vi "Drive_AutoShift.vi"(5 "Max":dbl format="%#_13g", 6 "Force Low Gear":bool, 7 "ShifterRef":T2={"DevStatus"={"status"=FALSE, "code"=0, "source"=""}, "Pneumatics Control Module"=0, "Forward Solenoid Channel"=enum."Invalid", "Reverse Solenoid Channel"=enum."Invalid"}, 8 "Right  Input":dbl, 9 "Left Input":dbl, 10 "Right RPM":dbl, 11 "Left RPM":dbl) -> (1 "Shifting":bool, 2 "Right Output":dbl, 3 "Left Output":dbl, 4 "Gear":T1)   [LabVIEW 2016]
uses:
  <vilib>/Rock Robotics/WPI/Solenoid/WPI_SolenoidDevRef.ctl
  <vilib>/Rock Robotics/WPI/Solenoid/WPI_SolenoidChannel.ctl
  <vilib>/Rock Robotics/WPI/Solenoid/WPI_SolenoidValue.ctl
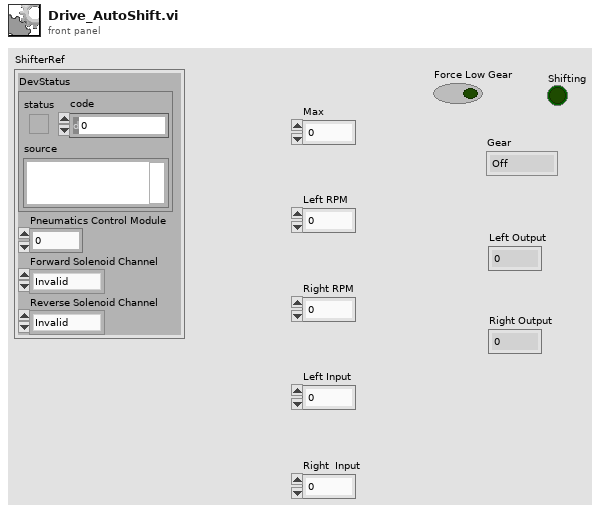
[diagram p1: front panel]
types:
  T1 = typedef "WPI_SolenoidValue.ctl" = enum16{"Off", "On", "Forward", "Reverse"}
  T2 = typedef "WPI_SolenoidDevRef.ctl" = cluster{"DevStatus":errorcluster, "Pneumatics Control Module":u8, "Forward Solenoid Channel":T3, "Reverse Solenoid Channel":T3}
  T3 = typedef "WPI_SolenoidChannel.ctl" = enum8{"Solenoid 0", "Solenoid 1", "Solenoid 2", "Solenoid 3", "Solenoid 4", "Solenoid 5", "Solenoid 6", "Solenoid 7", "Invalid"}
  T4 = cluster{"OutputMAX":dbl, "OutputMIN":dbl, "InputMAX":dbl, "InputMIN":dbl}
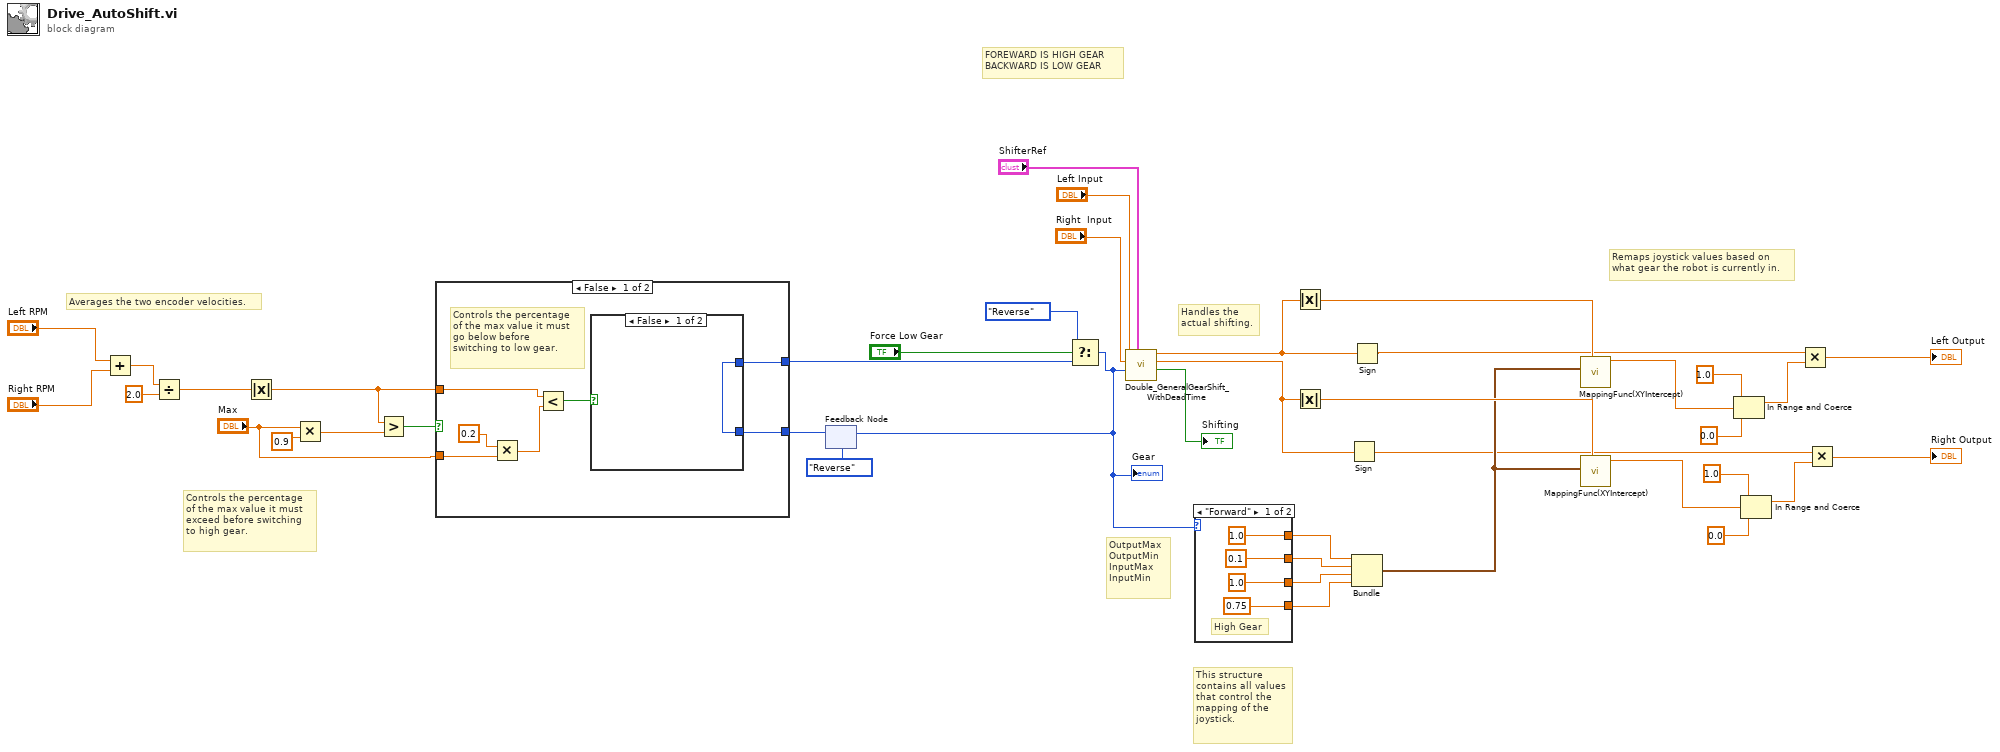
[diagram p0: block diagram]
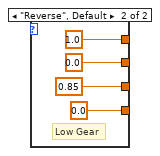
[diagram p2: hidden frame]
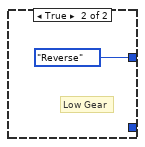
[diagram p3: hidden frame]
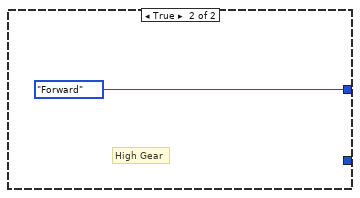
[diagram p4: hidden frame]
diagram:
  # "OutputMax\nOutputMin\nInputMax\nInputMin"
  # "This structure\ncontains all values\nthat control the\nmapping of the \njoystick."
  # "Remaps joystick values based on\nwhat gear the robot is currently in."
  # "Handles the\nactual shifting."
  # "FOREWARD IS HIGH GEAR\nBACKWARD IS LOW GEAR"
  # "Controls the percentage\nof the max value it must \nexceed before switching\nto high gear."
  # "Averages the two encoder velocities."
  n1 = Add(x="Left RPM", y="Right RPM") -> (x+y=w30:dbl)
  n2 = Divide(x=w30, y=2.0) -> (x/y=w7:dbl)
  n3 = Absolute Value(x=w7) -> (abs(x)=w6:dbl)
  n4 = Multiply(x="Max", y=0.9) -> (x*y=w40:dbl)
  n5 = Greater?(x=w6, y=w40) -> (0:w39:bool)
  n6 = feedback #1(WPI_SolenoidValue."Reverse" ("Shift Value")) -> (w3:T1)
  n7 = case shown="False" w39 {
    tunnel: [w44 WPI_SolenoidValue."Forward" ("Shift Value")] -> w21
    tunnel: "Max" -> [w47 _]
    tunnel: w3 -> [w43 _]
    tunnel: w6 -> [w42 _]
    frame False {
      # "Controls the percentage\nof the max value it must \ngo below before \nswitching to low gear."
      n8 = Multiply(x=0.2, y=w47) -> (x*y=w45:dbl)
      n9 = Less?(x=w42, y=w45) -> (x < y?=w48:bool)
      n10 = case shown="False" w48 {
        tunnel: [w49 WPI_SolenoidValue."Reverse" ("Shift Value")] -> w44
        tunnel: w43 -> [w49 _]
        frame False {
        }
        frame True {
          # "Low Gear"
        }
      }
    }
    frame True {
      # "High Gear"
    }
  }
  n11 = Select(t=WPI_SolenoidValue."Reverse", s="Force Low Gear", f=w21) -> (s? t:f=w2:T1)
  "Gear" <- w2
  n12 = feedback-in #1(w2) -> ()
  n13 = call "Double_GeneralGearShift_WithDeadTime.vi"("ShifterRef"="ShifterRef", "Shift Value"=w2, "Right"="Right  Input", "Left"="Left Input") -> ("Shifting"=→"Shifting":bool, "Right Output"=w15:dbl, "Left Output"=w13:dbl)  [unwired: 4 in, 1 out]
  n14 = case shown="\"Forward\"" w2 {
    tunnel: [1.0 ("OutputMAX") 1.0 ("OutputMAX")] -> w18
    tunnel: [0.1 ("OutputMIN") 0.0 ("OutputMIN")] -> w17
    tunnel: [1.0 ("InputMAX") 0.85 ("InputMAX")] -> w19
    tunnel: [0.75 ("InputMIN") 0.0 ("InputMIN")] -> w20
    frame "Forward" {
      # "High Gear"
    }
    frame "Reverse", Default {
      # "Low Gear"
    }
  }
  n15 = Absolute Value(x=w13) -> (abs(x)=w35:dbl)
  n16 = Absolute Value(x=w15) -> (abs(x)=w25:dbl)
  n17 = Sign(1:w15) -> (0:w14:dbl)
  n18 = Sign(1:w13) -> (0:w12:dbl)
  n19 = Bundle("OutputMAX"=w18, "OutputMIN"=w17, "InputMAX"=w19, "InputMIN"=w20) -> (w16:T4)  [unwired: 1 in]
  n20 = call "MappingFunc(XYIntercept).vi"("Input"=w35, "Cluster"=w16) -> ("Output"=w34:dbl)  [unwired: 9 in]
  n21 = call "MappingFunc(XYIntercept).vi"("Input"=w25, "Cluster"=w16) -> ("Output"=w26:dbl)  [unwired: 9 in]
  n22 = In Range and Coerce(upper limit=1.0, x=w34, lower limit=0.0) -> (coerced(x)=w31:dbl)  [unwired: 1 out]
  n23 = In Range and Coerce(upper limit=1.0, x=w26, lower limit=0.0) -> (coerced(x)=w27:dbl)  [unwired: 1 out]
  n24 = Multiply(x=w12, y=w31) -> (x*y=→"Left Output":dbl)
  n25 = Multiply(x=w14, y=w27) -> (x*y=→"Right Output":dbl)
